vi "Xiang move.vi"(1 "Color":i32, 2 "Array Position":cluster{"Row":i32, "Column":i32}, 3 "Chess Array":i32[][](array[numeric])=[[140, 130, 120, 110, 100, 111, 121, 131, 141], [-1, -1, -1, -1, -1, -1, -1, -1, -1], [-1, 150, -1, -1, -1, -1, -1, 151, -1], [160, -1, 161, -1, 162, -1, 163, -1, 164], [-1, -1, -1, -1, -1, -1, -1, -1, -1], [-1, -1, -1, -1, -1, -1, -1, -1, -1], [260, -1, 261, -1, 262, -1, 263, -1, 264], [-1, 250, -1, -1, -1, -1, -1, 251, -1], [-1, -1, -1, -1, -1, -1, -1, -1, -1], [240, 230, 220, 210, 200, 211, 221, 231, 241]]) -> (0 "Xiang move":cluster{i32, i32}[](array[cluster]))   [LabVIEW 2009]
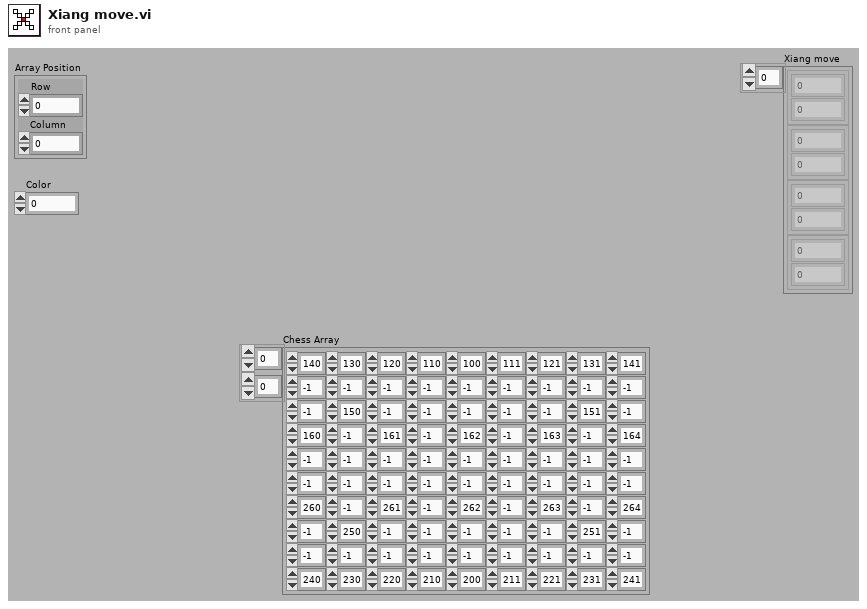
[diagram p1: front panel]
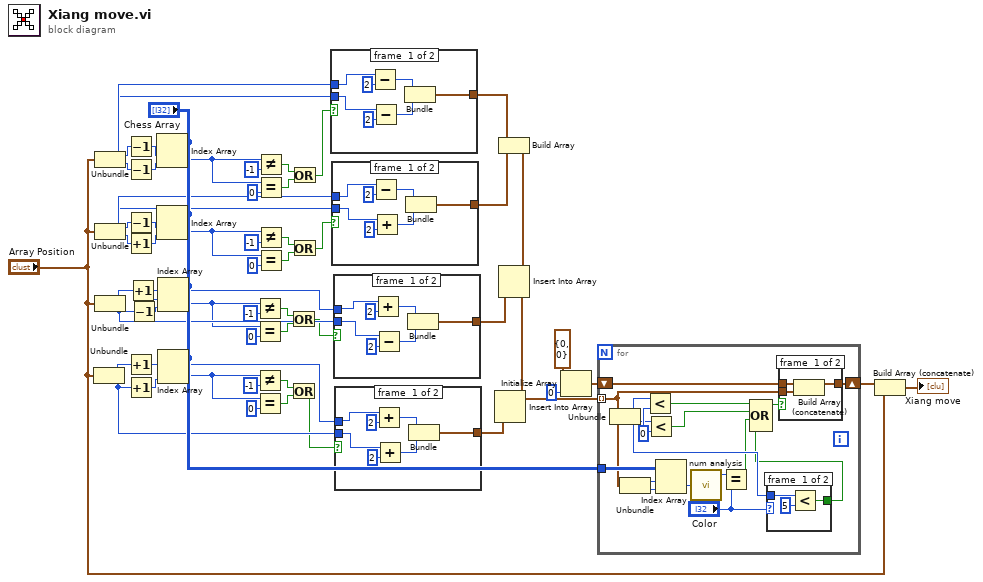
[diagram p0: block diagram]
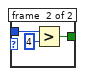
[diagram p2: hidden frame]
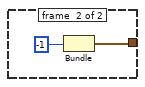
[diagram p4: hidden frame]
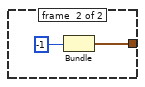
[diagram p5: hidden frame]
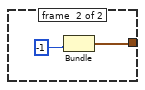
[diagram p6: hidden frame]
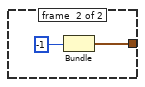
[diagram p7: hidden frame]
diagram:
  n1 = Unbundle("Array Position") -> ("Row"=w42:i32, "Column"=w48:i32)
  n2 = Unbundle("Array Position") -> ("Row"=w54:i32, "Column"=w51:i32)
  n3 = Unbundle("Array Position") -> ("Row"=w50:i32, "Column"=w46:i32)
  n4 = Unbundle("Array Position") -> ("Row"=w44:i32, "Column"=w49:i32)
  n5 = Decrement(x=w54) -> (x-1=w52:i32)
  n6 = Decrement(x=w51) -> (x-1=w13:i32)
  n7 = Decrement(x=w50) -> (x-1=w47:i32)
  n8 = Increment(x=w46) -> (x+1=w12:i32)
  n9 = Increment(x=w42) -> (x+1=w10:i32)
  n10 = Increment(x=w48) -> (x+1=w43:i32)
  n11 = Increment(x=w44) -> (x+1=w11:i32)
  n12 = Decrement(x=w49) -> (x-1=w45:i32)
  n13 = Index Array(array="Chess Array", index (row)=w52, index (col)=w13) -> (element=w40:i32)
  n14 = Index Array(array="Chess Array", index (row)=w47, index (col)=w12) -> (element=w30:i32)
  n15 = Index Array(array="Chess Array", index (row)=w11, index (col)=w45) -> (element=w21:i32)
  n16 = Index Array(array="Chess Array", index (row)=w10, index (col)=w43) -> (element=w20:i32)
  n17 = Not Equal?(x=w21, y=-1) -> (x != y?=w27:bool)
  n18 = Equal?(x=w21, y=0) -> (x = y?=w26:bool)
  n19 = Not Equal?(x=w20, y=-1) -> (x != y?=w24:bool)
  n20 = Equal?(x=w20, y=0) -> (x = y?=w25:bool)
  n21 = Not Equal?(x=w40, y=-1) -> (x != y?=w38:bool)
  n22 = Equal?(x=w40, y=0) -> (x = y?=w37:bool)
  n23 = Not Equal?(x=w30, y=-1) -> (x != y?=w34:bool)
  n24 = Equal?(x=w30, y=0) -> (x = y?=w35:bool)
  n25 = Or(x=w27, y=w26) -> (x .or. y?=w19:bool)
  n26 = Or(x=w24, y=w25) -> (x .or. y?=w18:bool)
  n27 = Or(x=w38, y=w37) -> (x .or. y?=w36:bool)
  n28 = Or(x=w34, y=w35) -> (x .or. y?=w31:bool)
  n29 = case shown="False" w36 {
    tunnel: w54 -> [w61 _]
    tunnel: w51 -> [w57 _]
    tunnel: [w55 w62] -> w9
    frame #0 {
      n30 = Subtract(x=w61, y=2) -> (x-y=w56:i32)
      n31 = Subtract(x=w57, y=2) -> (x-y=w59:i32)
      n32 = Bundle(w56, w59) -> (w55:cluster{i32, i32})  [unwired: 1 out]
    }
    frame #1 {
      w63 = -1 ("y")
      n33 = Bundle("y"=w63, "y"=w63) -> (w62:cluster{"y":i32, "y":i32})  [unwired: 1 out]
    }
  }
  n34 = case shown="False" w31 {
    tunnel: w50 -> [w70 _]
    tunnel: w46 -> [w66 _]
    tunnel: [w64 w71] -> w8
    frame #0 {
      n35 = Subtract(x=w70, y=2) -> (x-y=w65:i32)
      n36 = Add(x=w66, y=2) -> (x+y=w68:i32)
      n37 = Bundle(w65, w68) -> (w64:cluster{i32, i32})  [unwired: 1 out]
    }
    frame #1 {
      w72 = -1 ("y")
      n38 = Bundle("y"=w72, "y"=w72) -> (w71:cluster{"y":i32, "y":i32})  [unwired: 1 out]
    }
  }
  n39 = case shown="False" w19 {
    tunnel: w44 -> [w77 _]
    tunnel: w49 -> [w76 _]
    tunnel: [w73 w80] -> w6
    frame #0 {
      n40 = Add(x=w77, y=2) -> (x+y=w75:i32)
      n41 = Subtract(x=w76, y=2) -> (x-y=w74:i32)
      n42 = Bundle(w75, w74) -> (w73:cluster{i32, i32})  [unwired: 1 out]
    }
    frame #1 {
      w81 = -1 ("y")
      n43 = Bundle("y"=w81, "y"=w81) -> (w80:cluster{"y":i32, "y":i32})  [unwired: 1 out]
    }
  }
  n44 = case shown="False" w18 {
    tunnel: w42 -> [w86 _]
    tunnel: w48 -> [w85 _]
    tunnel: [w82 w89] -> w4
    frame #0 {
      n45 = Add(x=w86, y=2) -> (x+y=w84:i32)
      n46 = Add(x=w85, y=2) -> (x+y=w83:i32)
      n47 = Bundle(w84, w83) -> (w82:cluster{i32, i32})  [unwired: 1 out]
    }
    frame #1 {
      w90 = -1 ("y")
      n48 = Bundle("y"=w90, "y"=w90) -> (w89:cluster{"y":i32, "y":i32})  [unwired: 1 out]
    }
  }
  n49 = Build Array(w9, w8) -> (w7:cluster{"y":i32, "y":i32}[])
  n50 = Insert Into Array(array=w7, new element=w6) -> (w5:cluster{"y":i32, "y":i32}[])  [unwired: 1 in]
  n51 = Insert Into Array(array=w5, new element=w4) -> (w17:cluster{"y":i32, "y":i32}[])  [unwired: 1 in]
  n52 = Initialize Array(cluster{i32, i32} {0, 0} ("Output Cluster"), 0 ("Dimension Size")) -> (w16:cluster{i32, i32}[])
  n53 = for {
    tunnel: w17 -> [w95] mode=indexing
    shift-right: [w102] -> w3
    shift-left: w16 -> [w103]
    tunnel: "Chess Array" -> [w101]
    w107 = 0 ("y")
    n54 = Unbundle(w95) -> ("y"=w94:i32, "y"=w98:i32)
    n55 = Unbundle(w95) -> ("y"=w97:i32, "y"=w96:i32)
    n56 = Less?(x=w94, y=w107) -> (x < y?=w105:bool)
    n57 = Less?(x=w98, y=w107) -> (x < y?=w106:bool)
    n58 = Index Array(array=w101, index (row)=w97, index (col)=w96) -> (element=w100:i32)
    n59 = call "num analysis.vi"("x"=w100) -> ("Color"=w99:i32)  [unwired: 2 out]
    n60 = Equal?(x=w99, y="Color") -> (x = y?=w92:bool)
    n61 = case shown="1, Default" "Color" {
      tunnel: w94 -> [w109 w112]
      tunnel: [w108 w111] -> w91
      frame #0 {
        n62 = Less?(x=w109, y=5) -> (x < y?=w108:bool)
      }
      frame #1 {
        n63 = Greater?(x=w112, y=4) -> (0:w111:bool)
      }
    }
    n64 = Compound Arithmetic op=OR(w105, w106, w92, w91) -> (w104:bool)
    n65 = case shown="False" w104 {
      tunnel: w103 -> [w116 w117]
      tunnel: [w115 w117] -> w102
      tunnel: w95 -> [w114 _]
      frame #0 {
        n66 = Build Array (concatenate)(w116, w114) -> (w115:cluster{"y":i32, "y":i32}[])
      }
      frame #1 {
      }
    }
  }
  n67 = Build Array (concatenate)(w3, "Array Position") -> (→"Xiang move":cluster{"Row":i32, "Column":i32}[])
